vi "Actor Core.vi"(8 "error in":errorcluster, 11 "Client in":refnum<class "Client.lvclass">) -> (0 "error out":errorcluster, 3 "Actor out":refnum<class "Actor.lvclass">)   [LabVIEW 2021, in "Client.lvlib" / "Client.lvclass"]
doc: "(<B>Filename</B>: Actor Framework.lvlib:Actor.lvclass:Actor Core.vi)\n\nReceives messages to the actor, reacts to them, and initiates any error handling that may shut the actor down.\n\nDescendant classes may override this VI to append parallel tasks for the actor to complete while it handles messages. Overrides use the Call Parent Class Method node."
uses:
  Client.lvclass
  C:/Program Files/National Instruments/LabVIEW 2021/vi.lib/ActorFramework/Actor/Actor.lvclass
  <vilib>/ActorFramework/Actor/Actor.lvclass
  Client.lvclass/Client.ctl
  <vilib>/ActorFramework/Actor/Actor.lvclass/Actor.ctl
  <vilib>/ActorFramework/Message Enqueuer/Message Enqueuer.lvclass/Message Enqueuer.ctl
  <vilib>/ActorFramework/Message Enqueuer/Init from Existing Queue.vi
  <vilib>/ActorFramework/Message Enqueuer/Enqueue.vi
  Client Messages/ConnectToServer Msg/ConnectToServer Msg.lvclass
  C:/Program Files/National Instruments/LabVIEW 2021/vi.lib/ActorFramework/Message/Message.lvclass
  <vilib>/ActorFramework/Stop Msg/Stop Msg.lvclass
  Interfaces/Chatter/Chatter Messages/SendChatMsg Msg/SendChatMsg Msg.lvclass
  <vilib>/ActorFramework/Message Priority Queue/Priority Enqueue.vi
  <vilib>/ActorFramework/Message Enqueuer/Message Enqueuer.lvclass
panel:
  in  "SendBtn":bool
  in  "MsgToSendStr":string
  out "ChatStr":string caption="Chat:"
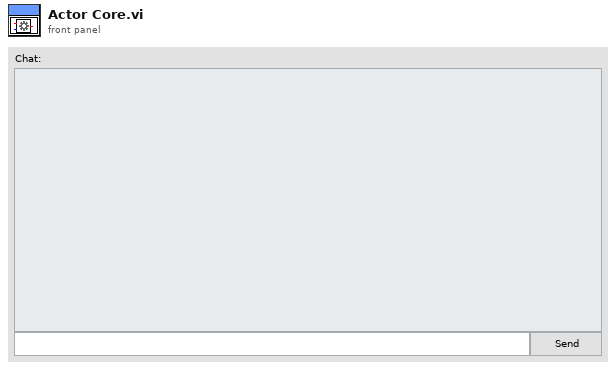
[diagram p1: front panel]
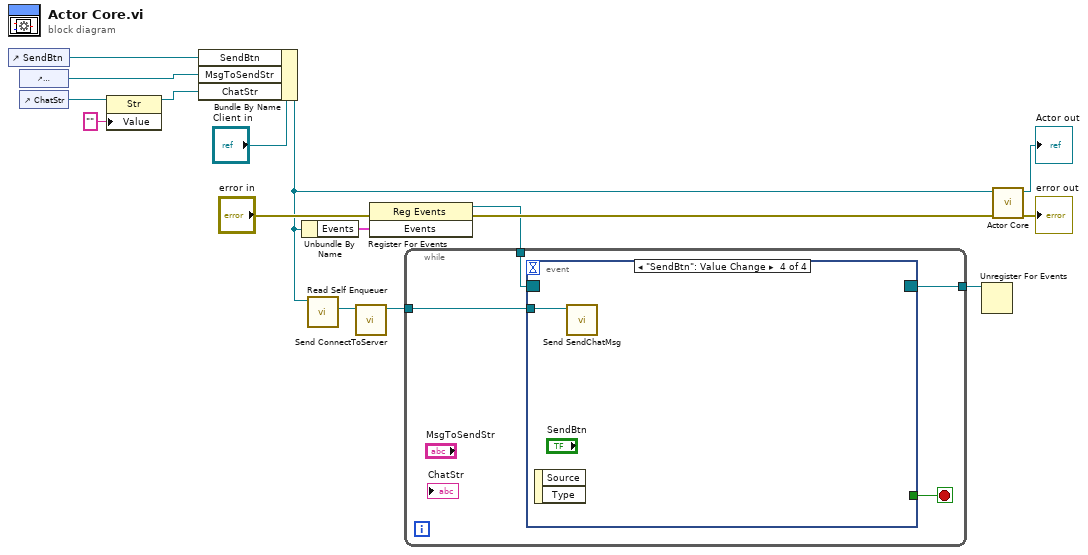
[diagram p0: block diagram]
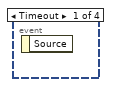
[diagram p2: hidden frame]
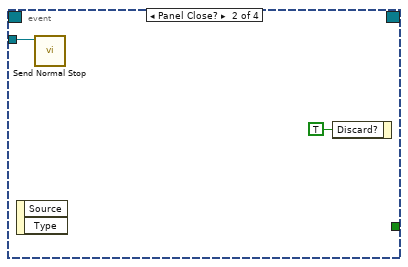
[diagram p3: hidden frame]
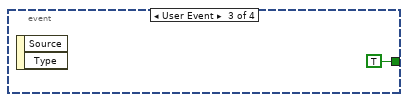
[diagram p4: hidden frame]
diagram:
  n1 = control-ref of="SendBtn"() -> (w12:refnum<vi>)
  n2 = control-ref of="MsgToSendStr"() -> (w11:refnum<vi>)
  n3 = control-ref of="ChatStr"() -> (w10:refnum<vi>)
  n4 = property class="Str"(reference=w10, "Value"="") -> (reference out=w2:refnum<vi>)  [unwired: 1 in, 1 out]
  n5 = Bundle By Name(cluster="Client in", "SendBtn"=w12, "MsgToSendStr"=w11, "ChatStr"=w2) -> (w5:refnum<class "Client.lvclass">)
  n6 = Unbundle By Name(w5) -> ("Events"=w8:cluster{"Stop":refnum<user-event>})
  n7 = call <vilib>:"Read Self Enqueuer.vi"("Actor"=w5) -> ("Self Enqueuer"=w4:refnum<class "Message Enqueuer.lvclass">)  [unwired: 10 in]
  n8 = call "Send ConnectToServer.vi"("Message Enqueuer"=w4) -> ("Message Enqueuer out"=w3:refnum<class "Message Enqueuer.lvclass">)  [unwired: 9 in, 1 out]
  n9 = register-events(error in="error in", w8) -> (reference out=w7:refnum<event-registration>, error out=w9:errorcluster)  [unwired: 1 in]
  n10 = while {
    tunnel: w7 -> [w20]
    tunnel: [w19] -> w6
    tunnel: w3 -> [w18]
    stop <- w17 stop-if-true
    n11 = event shown="[3] \"SendBtn\": Value Change" {
      selector: w20 -> [_ _ _ _]
      dyn-events: [_ _ _ _] -> w19
      timeout: _ -> [_ _ _ _]
      tunnel: w18 -> [_ w21 _ w24]
      tunnel: [_ _ TRUE _] -> w17
      event Timeout {
        n12 = event-data() -> ()  [unwired: 1 in, 1 out]
      }
      event Panel Close? {
        n13 = event-data() -> ()  [unwired: 1 in, 2 out]
        n14 = call <vilib>:"Send Normal Stop.vi"("Message Enqueuer"=w21) -> ()  [unwired: 10 in, 1 out]
        n15 = event-data("Discard?"=TRUE) -> ()  [unwired: 1 in, 1 out]
      }
      event User Event {
        n16 = event-data() -> ()  [unwired: 1 in, 2 out]
      }
      event "SendBtn": Value Change {
        n17 = event-data() -> ()  [unwired: 1 in, 2 out]
        n18 = call "Send SendChatMsg.vi"("Message Enqueuer"=w24) -> ()  [unwired: 9 in, 2 out]
      }
    }
  }
  n19 = Unregister For Events(event registration refnum=w6) -> ()  [unwired: 1 in, 1 out]
  n20 = call-parent "Actor Core.vi"("error in"=w9, "Actor in"=w5) -> ("error out"=→"error out":errorcluster, "Actor out"=→"Actor out":refnum<class "Actor.lvclass">)  [unwired: 8 in]
